vi "getVerticalChannelSettingsFromHW.vi"(8 "error in (no error)":errorcluster, 11 "TektronixDPO in":refnum<class "TektronixDPO.lvclass">) -> (0 "error out":errorcluster, 3 "TektronixDPO out":refnum<class "TektronixDPO.lvclass">)   [LabVIEW 2013, in "TektronixDPO.lvclass"]
uses:
  TektronixDPO.lvclass
  TektronixDPO.lvclass/TektronixDPO.ctl
  SupportClasses/TektronixDPOPhysicalDevice/TektronixDPO_PhysicalDevice.lvclass
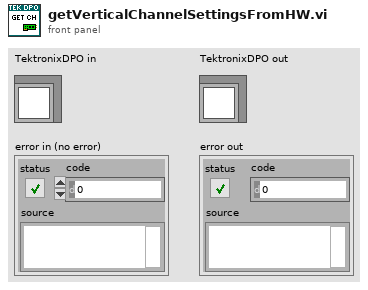
[diagram p1: front panel]
types:
  T1 = typedef "Choices.lvlib/Choice80.ctl" = u16
  T2 = cluster{"Channel":T1, "offset":dbl, "verticalrange":dbl, "Impedance":u16, "Probe Attenuation":dbl, "Vertical Coupling":u16, "Bandwidth":u16, "Enabled":bool}
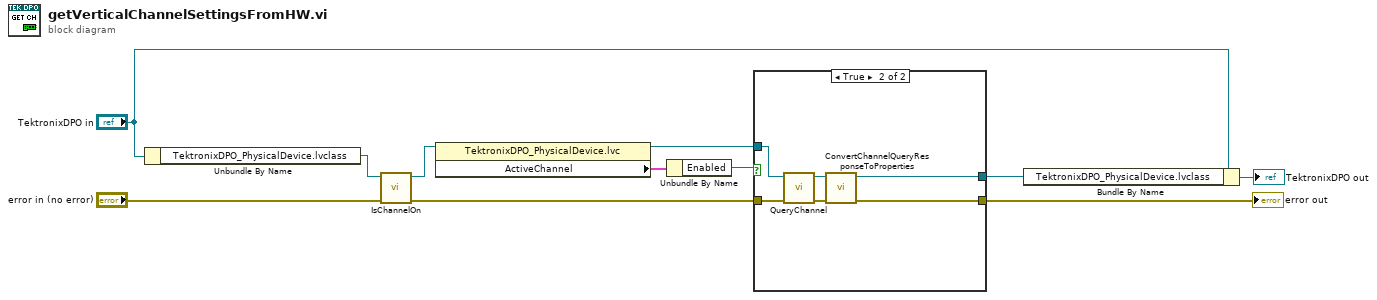
[diagram p0: block diagram]
diagram:
  n1 = Unbundle By Name("TektronixDPO in") -> ("TektronixDPO_PhysicalDevice.lvclass"=w8:refnum<class "TektronixDPO_PhysicalDevice.lvclass">)
  n2 = call "IsChannelOn.vi"("error in (no error)"="error in (no error)", "TektronixDPO_PhysicalDevice in"=w8) -> ("error out"=w9:errorcluster, "TektronixDPO_PhysicalDevice out"=w6:refnum<class "TektronixDPO_PhysicalDevice.lvclass">)  [unwired: 8 in]
  n3 = property class="TektronixDPO_PhysicalDevice.lvc"(reference=w6) -> (reference out=w3:refnum<class "TektronixDPO_PhysicalDevice.lvclass">, "ActiveChannel"=w5:T2)  [unwired: 1 in, 1 out]
  n4 = Unbundle By Name(w5) -> ("Enabled"=w4:bool)
  n5 = case shown="True" w4 {
    tunnel: [w12 w19] -> w2
    tunnel: [w13 w18] -> w1
    tunnel: w9 -> [w13 w16]
    tunnel: w3 -> [w12 w14]
    frame False {
    }
    frame True {
      n6 = call "QueryChannel.vi"("error in (no error)"=w16, "TektronixDPO_PhysicalDevice in"=w14) -> ("error out"=w17:errorcluster, "TektronixDPO_PhysicalDevice out"=w15:refnum<class "TektronixDPO_PhysicalDevice.lvclass">)  [unwired: 8 in]
      n7 = call-dynamic "ConvertChannelQueryResponseToProperties.vi"("error in (no error)"=w17, "TektronixDPO_PhysicalDevice.lvclass"=w15) -> ("error out"=w18:errorcluster, "TektronixDPO_PhysicalDevice.lvclassOut"=w19:refnum<class "TektronixDPO_PhysicalDevice.lvclass">)  [unwired: 8 in]
    }
  }
  "error out" <- w1
  n8 = Bundle By Name(cluster="TektronixDPO in", "TektronixDPO_PhysicalDevice.lvclass"=w2) -> (→"TektronixDPO out":refnum<class "TektronixDPO.lvclass">)
